vi "Test App Remove Process Before Start Returns Error.vi"(8 "error in (no error)":errorcluster, 11 "Rig Test in":refnum<class "Application Dev Test.lvclass">) -> (0 "error out":errorcluster, 3 "Rig Test out":refnum<class "Application Dev Test.lvclass">)   [LabVIEW 2020, in "Application Dev Test.lvclass"]
uses:
  Application Dev Test.lvclass
  C:/Program Files (x86)/National Instruments/LabVIEW 2020/vi.lib/Astemes/LUnit/Test Case.lvclass
  source/Framework/Process/Process.lvclass
  source/Framework/Process/Process.lvclass/Process.ctl
  source/Framework/Application/Application.lvclass/Application.ctl
  <vilib>/Astemes/LUnit/Test Case.lvclass/Test Case.ctl
  source/Framework/Application/Private/Add Process to Map.vi
  source/Framework/Application/Private/Throw Error If Process Already in App.vi
  source/Framework/Process/Protected/Messaging/Send Message.vi
  source/Framework/Process/Public/Lifecycle/Get Lifecycle State.vi
  source/Framework/Process/Protected/SubVIs/Set Context.vi
  source/Framework/Application/Private/Remove Process from App.vi
  source/Framework/Application/Private/Parse Process Name.vi
  source/Framework/Application/Private/Remove Process from Map.vi
  source/Framework/Process/Protected/SubVIs/Clear Context.vi
  <vilib>/Astemes/LUnit/Palette/Fail.vi
  <vilib>/Astemes/LUnit/Palette/Pass.vi
  <vilib>/Astemes/LUnit/Set Assertion Type.vi
  source/Framework/Application/Public/Get Process.vi
  source/Framework/Process/Private/SubVIs/Handle Debug Data.vi
  <vilib>/Utility/error.llb/Clear Errors.vi
  source/Framework/Process/Public/Lifecycle/Leave Process Loop.vi
  source/Framework/Process/Protected/Messaging/Request Message.vi
  <vilib>/AdvancedString/Delimited String to 1D String Array.vi
  <vilib>/Astemes/LUnit/Add test result.vi
  source/Framework/Application/Private/Retrieve Process from App.vi
  source/Framework/Application/Private/Get Process from Map.vi
  source/Framework/Logging/Log Debug.vi
  <vilib>/AdvancedString/1D String Array to Delimited String.vi
  <vilib>/Utility/High Resolution Relative Seconds.vi
  source/Framework/Process/Private/SubVIs/Enqueue Request Message.vi
  <vilib>/Astemes/LUnit/LUnit Record Assertion Result.vi
  <vilib>/Astemes/LUnit/LUnit Aggregate Assertion Results.vi
  <vilib>/Astemes/LUnit/Method Result/LUnit Merge Status.vi
  <vilib>/Astemes/LUnit/LUnit Concatenate result strings.vi
  source/Framework/Application/Application.lvclass
  C:/Git/astemes-triarc-framework/source/Framework/Process/Process.lvclass
  <vilib>/Utility/error.llb/Error Cluster From Error Code.vi
  source/Framework/Process/Public/Read Name.vi
  source/Framework/Process/Private/SubVIs/Wait for Response Message.vi
  <vilib>/Astemes/LUnit/Test Case.lvclass
panel:
  out "error out 2":errorcluster
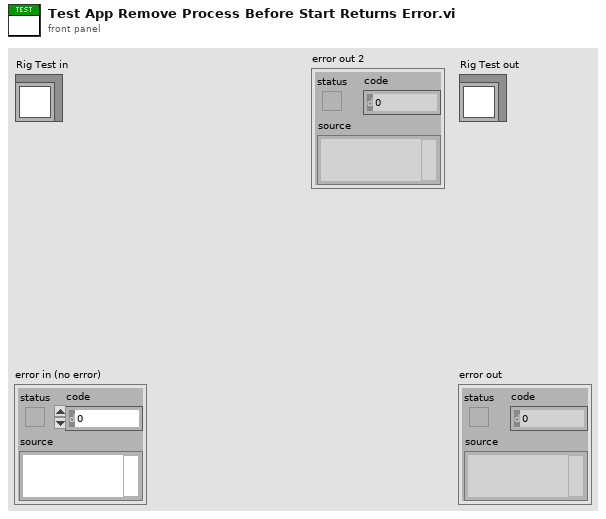
[diagram p1: front panel]
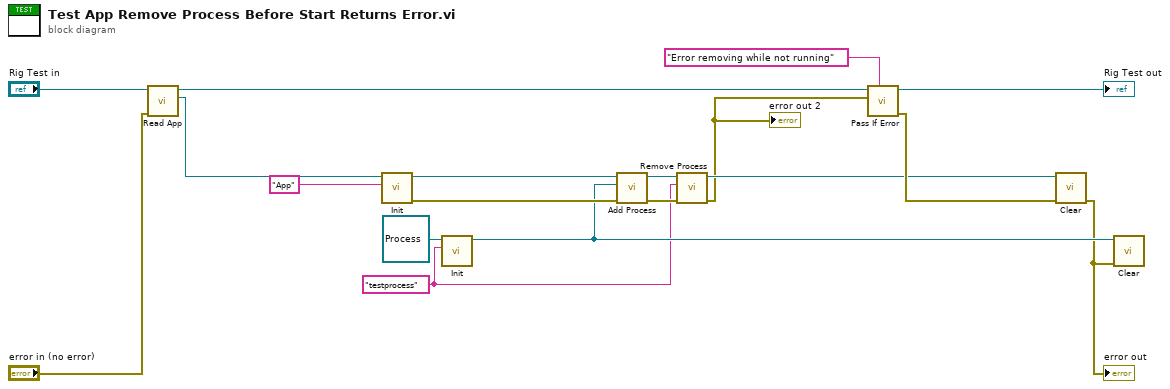
[diagram p0: block diagram]
diagram:
  w2 = "testprocess" ("Name")
  n1 = call "Read App.vi"("error in (no error)"="error in (no error)", "Application Test In"="Rig Test in") -> ("App out"=w17:refnum<class "Application.lvclass">, "Application Test Out"=w8:refnum<class "Application Dev Test.lvclass">)  [unwired: 7 in, 1 out]
  n2 = call-dynamic "Init.vi"("Name"="App", "Process In"=w17) -> ("error out"=w9:errorcluster, "Process Out"=w10:refnum<class "Application.lvclass">)  [unwired: 8 in]
  n3 = call-dynamic "Init.vi"("Name"=w2, "Process In"=refnum<class "Process.lvclass"> refnum ("Process.lvclass")) -> ("Process Out"=w4:refnum<class "Process.lvclass">)  [unwired: 8 in, 1 out]
  n4 = call "Add Process.vi"("error in (no error)"=w9, "Process"=w4, "Application In"=w10) -> ("error out"=w14:errorcluster, "Application Out"=w6:refnum<class "Application.lvclass">)  [unwired: 7 in]
  n5 = call "Remove Process.vi"("error in (no error)"=w14, "Process Name"=w2, "Application In"=w6) -> ("error out"=w1:errorcluster, "Application Out"=w5:refnum<class "Application.lvclass">)  [unwired: 6 in, 1 out]
  "error out 2" <- w1
  n6 = call <vilib>:"Pass If Error.vi"("Description"="Error removing while not running", "Assert error"=w1, "LUnit Test Case In"=w8) -> ("error out"=w12:errorcluster, "LUnit Test Case Out"=→"Rig Test out":refnum<class "Application Dev Test.lvclass">)  [unwired: 7 in]
  n7 = call-dynamic "Clear.vi"("error in (no error)"=w12, "Application In"=w5) -> ("error out"=w3:errorcluster)  [unwired: 9 in]
  "error out" <- w3
  n8 = call-dynamic "Clear.vi"("error in (no error)"=w3, "Process In"=w4) -> ()  [unwired: 9 in, 1 out]
